vi "HXG2_Pre-Write.vi"(8 "error in (no error)":errorcluster, 10 "EXVs Multiplier":dbl, 11 "PID Ctrls":T1) -> (0 "error out":errorcluster, 2 "Analog Ctrl Out":dbl[](array[numeric]))   [LabVIEW 2012]
uses:
  Controls/HXG2_PIDctrlsOUT.ctl
  Modules/EnableAirGly/HXG2enable.ctl
panel:
  # "BlowerVFD"
  # "PumpVFD"
  # "ByPass Damper"
  # "AirHTR SCR"
  # "EXV Air Evap"
  # "GlyHTR SCR"
  # "EXV Gly Evap"
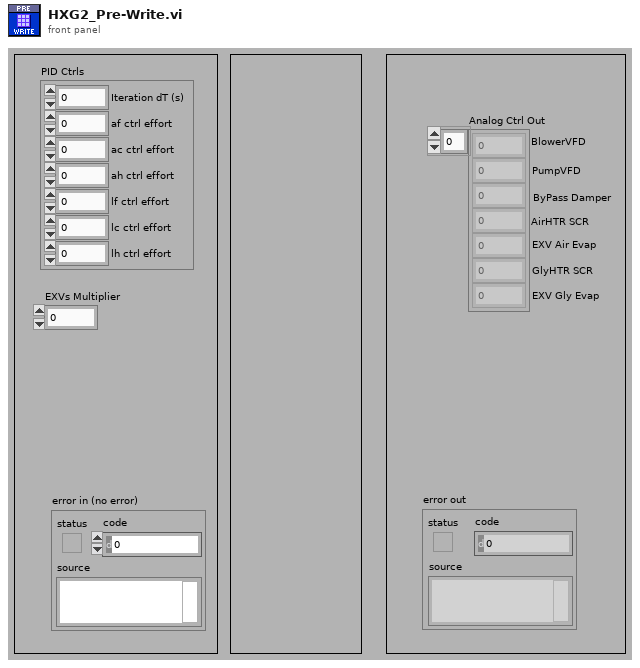
[diagram p1: front panel]
types:
  T1 = typedef "HXG2_PIDctrlsOUT.ctl" = cluster{"Iteration dT (s)":dbl, "af ctrl effort":dbl, "ac ctrl effort":dbl, "ah ctrl effort":dbl, "lf ctrl effort":dbl, "lc ctrl effort":dbl, "lh ctrl effort":dbl}
  T2 = typedef "HXG2enable.ctl" = enum16{"Write Refs", "Write", "Pass"}
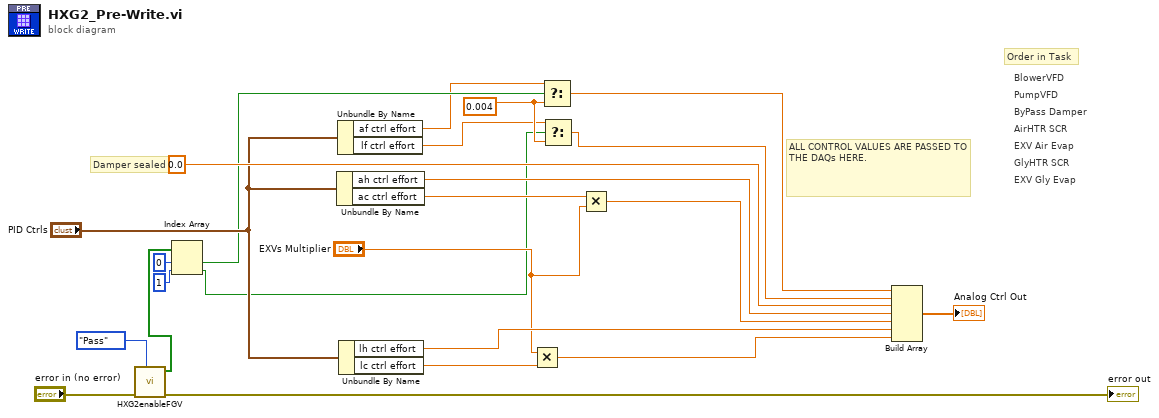
[diagram p0: block diagram]
diagram:
  w4 = 0.004 ("f")
  # "Damper sealed"
  # "Order in Task"
  # "EXV Gly Evap"
  # "GlyHTR SCR"
  # "EXV Air Evap"
  # "AirHTR SCR"
  # "ByPass Damper"
  # "PumpVFD"
  # "BlowerVFD"
  # "ALL CONTROL VALUES ARE PASSED TO\nTHE DAQs HERE."
  n1 = call "HXG2enableFGV.vi"("ENABLE Ctrl"=HXG2enable."Pass", "error in (no error)"="error in (no error)") -> ("error out"=→"error out":errorcluster, "Air-Liq Out"=w8:bool[])  [unwired: 7 in, 1 out]
  n2 = Index Array(array=w8, index #1=0 ("index"), index #2=1 ("index")) -> (element #1=w7:bool, element #2=w3:bool)
  n3 = Unbundle By Name("PID Ctrls") -> ("ah ctrl effort"=w14:dbl, "ac ctrl effort"=w15:dbl)
  n4 = Unbundle By Name("PID Ctrls") -> ("af ctrl effort"=w6:dbl, "lf ctrl effort"=w2:dbl)
  n5 = Unbundle By Name("PID Ctrls") -> ("lh ctrl effort"=w22:dbl, "lc ctrl effort"=w20:dbl)
  n6 = Multiply(x="EXVs Multiplier", y=w20) -> (x*y=w21:dbl)
  n7 = Select(t=w6, s=w7, f=w4) -> (s? t:f=w5:dbl)
  n8 = Select(t=w2, s=w3, f=w4) -> (s? t:f=w1:dbl)
  n9 = Multiply(x=w15, y="EXVs Multiplier") -> (x*y=w23:dbl)
  n10 = Build Array(w5, w1, 0.0 ("Damper Ctrl"), w14, w23, w22, w21) -> (→"Analog Ctrl Out":dbl[])
